vi "Autonomous Global Data.vi"() -> ()   [LabVIEW 2012]
panel:
  in  "Delay (sec)":dbl
  in  "Mode":u16(ring) items=["A", "B", "C", "D"]
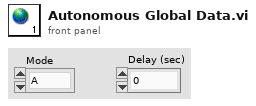
[diagram p1: front panel]
diagram:
